vi "Define DataTable Columns.vi"(8 "error in (no error)":errorcluster, 9 "ReadOnly":bool, 10 "ColumnSetup":T1[](array[typedef]) {"MinWidth" min=2 step=1; "AutoSizeMode" items=["None"=1, "ColumnHeader"=2, "AllCellsExceptHeader"=4, "AllCells"=6, "DisplayedCellsExceptHeader"=8, "DisplayedCells"=10, "Fill"=16]; "FillWeight" min=1 max=100}, 11 "DataTable In":refnum<class "DataTable.lvclass">) -> (0 "error out":errorcluster, 3 "DataTable Out":refnum<class "DataTable.lvclass">)   [LabVIEW 2020, in "DataGrid.lvlib" / "DataTable.lvclass"]
doc: "Defines the columns of the dataTable that is used to store all display data. If called more than once, it will add columns to the existing dataTable, so resulting in more (possibly duplicate) columns."
uses:
  DataTable/DataTable.lvclass
  GridColumn/ColumnDefinition.ctl
  GridColumn/ColumnType.ctl
  DataTable/DataTable.lvclass/DataTable.ctl
  System.Data
  DataTable/Read DataTable.vi
  GridColumn/GridColumn.lvclass
panel:
  out "fl":bool
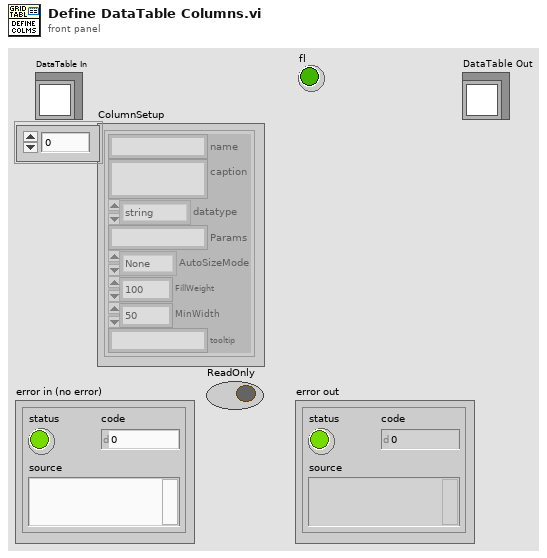
[diagram p1: front panel]
types:
  T1 = typedef "DataGrid.lvlib/GridColumn.lvclass/ColumnDefinition.ctl" = cluster{"name":string, "caption":string, "datatype":T2, "Params":string, "AutoSizeMode":i32, "FillWeight":sgl, "MinWidth":u32, "tooltip":string}
  T2 = typedef "DataGrid.lvlib/GridColumn.lvclass/ColumnType.ctl" = enum16{"string", "image", "check", "numeric", "timestamp", "button", "combo", "link"}
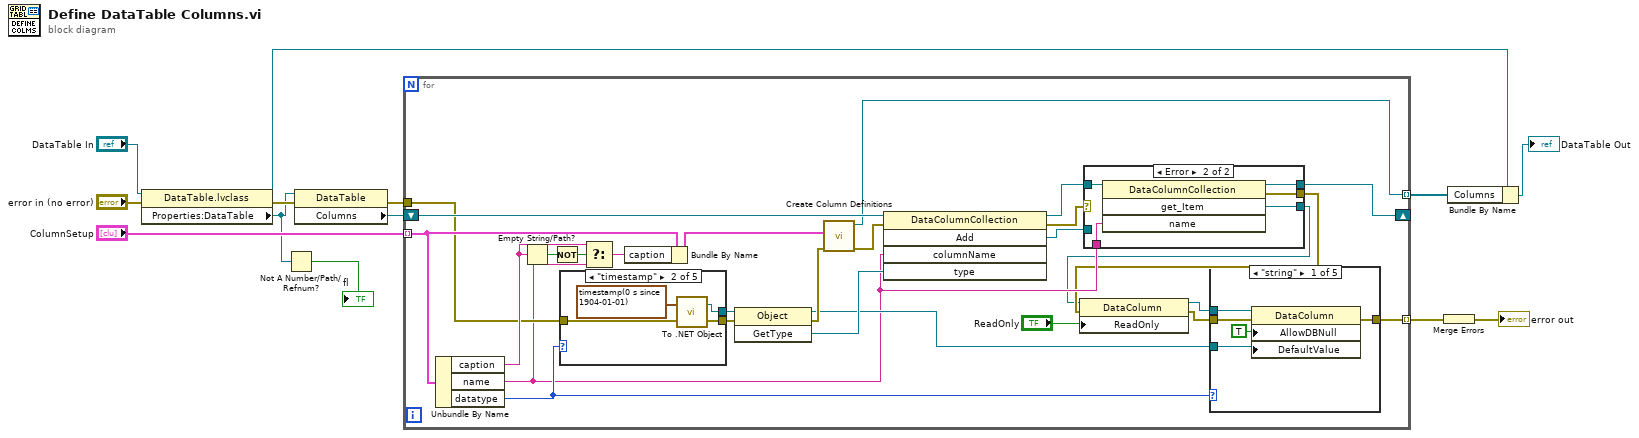
[diagram p0: block diagram]
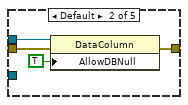
[diagram p3: hidden frame]
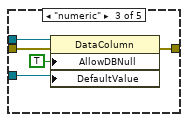
[diagram p4: hidden frame]
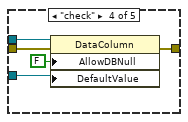
[diagram p5: hidden frame]
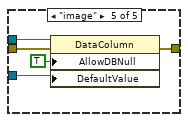
[diagram p6: hidden frame]
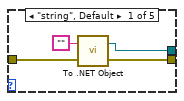
[diagram p7: hidden frame]
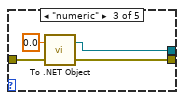
[diagram p8: hidden frame]
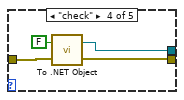
[diagram p9: hidden frame]
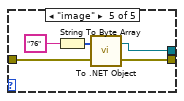
[diagram p10: hidden frame]
diagram:
  n1 = property class="DataTable.lvclass"(reference="DataTable In", error in="error in (no error)") -> (reference out=w8:refnum<class "DataTable.lvclass">, error out=w4:errorcluster, "Properties:DataTable"=w2:refnum<k24>)
  n2 = Not A Number/Path/Refnum?(number/path/refnum=w2) -> (NaN/Path/Refnum?=→"fl":bool)
  n3 = property class="DataTable"(reference=w2, error in=w4) -> (error out=w3:errorcluster, "Columns"=w10:refnum<k24>)  [unwired: 1 out]
  n4 = for {
    tunnel: "ColumnSetup" -> [w35] mode=indexing
    tunnel: [w40] -> w11 mode=indexing
    shift-right: [w16] -> _
    shift-left: w10 -> [w39]
    tunnel: [w38] -> w6 mode=indexing
    tunnel: w3 -> [w23]
    n5 = Unbundle By Name(w35) -> ("caption"=w33:string, "name"=w20:string, "datatype"=w22:T2)
    n6 = Empty String/Path?(string/path=w33) -> (empty?=w37:bool)
    n7 = Not(x=w37) -> (.not. x?=w24:bool)
    n8 = case shown="\"timestamp\"" w22 {
      tunnel: [w75 w79 w83 w87 w91] -> w31
      tunnel: [w74 w78 w82 w86 w90] -> w29
      tunnel: w23 -> [w73 w77 w81 w85 w89]
      frame "string", Default {
        n9 = call <vilib>:"To .NET Object.vi"("error in (no error)"=w73, "anything"="" ("name")) -> ("error out"=w74:errorcluster, ".NET object"=w75:refnum<k24>)
      }
      frame "timestamp" {
        n10 = call <vilib>:"To .NET Object.vi"("error in (no error)"=w77, "anything"=timestamp(0 s since 1904-01-01) ("name")) -> ("error out"=w78:errorcluster, ".NET object"=w79:refnum<k24>)
      }
      frame "numeric" {
        n11 = call <vilib>:"To .NET Object.vi"("error in (no error)"=w81, "anything"=0.0 ("name")) -> ("error out"=w82:errorcluster, ".NET object"=w83:refnum<k24>)
      }
      frame "check" {
        n12 = call <vilib>:"To .NET Object.vi"("error in (no error)"=w85, "anything"=FALSE) -> ("error out"=w86:errorcluster, ".NET object"=w87:refnum<k24>)
      }
      frame "image" {
        n13 = String To Byte Array(string="76") -> (unsigned byte array=w93:u8[])
        n14 = call <vilib>:"To .NET Object.vi"("error in (no error)"=w89, "anything"=w93) -> ("error out"=w90:errorcluster, ".NET object"=w91:refnum<k24>)
      }
    }
    n15 = Select(t=w33, s=w24, f=w20) -> (s? t:f=w36:string)
    n16 = Bundle By Name(cluster=w35, "caption"=w36) -> (w34:T1)
    n17 = invoke class="Object" method="GetType"(reference=w31, error in=w29) -> (reference out=w25:refnum<k24>, error out=w28:errorcluster, "GetType"=w30:refnum<k24>)  [unwired: 1 in]
    n18 = call "Create Column Definitions.vi"("error in (no error)"=w28, "Column"=w34) -> ("error out"=w21:errorcluster, "GridColumn out"=w38:refnum<class "GridColumn.lvclass">)  [unwired: 8 in]
    n19 = invoke class="DataColumnCollection" method="Add"(reference=w39, error in=w21, "columnName"=w20, "type"=w30) -> (reference out=w17:refnum<k24>, error out=w19:errorcluster, "Add"=w15:refnum<k24>)  [unwired: 1 in, 2 out]
    n20 = case shown="Error" w19 {
      selector: w19 -> [w43 _]
      tunnel: w17 -> [w41 w48]
      tunnel: [w42 w47] -> w14
      tunnel: w20 -> [_ w46]
      tunnel: [w43 w45] -> w18
      tunnel: [w41 w44] -> w16
      tunnel: w15 -> [w42 _]
      frame No Error {
      }
      frame Error {
        n21 = invoke class="DataColumnCollection" method="get_Item"(reference=w48, "name"=w46) -> (reference out=w44:refnum<k24>, error out=w45:errorcluster, "get_Item"=w47:refnum<k24>)  [unwired: 2 in, 1 out]
      }
    }
    n22 = property class="DataColumn"(reference=w14, error in=w18, "ReadOnly"="ReadOnly") -> (reference out=w27:refnum<k24>, error out=w26:errorcluster)
    n23 = case shown="\"string\"" w22 {
      tunnel: w27 -> [w51 w55 w60 w65 w70]
      tunnel: w26 -> [w53 w57 w62 w67 w72]
      tunnel: [w52 w56 w61 w66 w71] -> w40
      tunnel: w25 -> [w49 _ w58 w63 w68]
      frame "string" {
        n24 = property class="DataColumn"(reference=w51, error in=w53, "AllowDBNull"=TRUE, "DefaultValue"=w49) -> (error out=w52:errorcluster)  [unwired: 1 out]
      }
      frame Default {
        n25 = property class="DataColumn"(reference=w55, error in=w57, "AllowDBNull"=TRUE) -> (error out=w56:errorcluster)  [unwired: 1 out]
      }
      frame "numeric" {
        n26 = property class="DataColumn"(reference=w60, error in=w62, "AllowDBNull"=TRUE, "DefaultValue"=w58) -> (error out=w61:errorcluster)  [unwired: 1 out]
      }
      frame "check" {
        n27 = property class="DataColumn"(reference=w65, error in=w67, "AllowDBNull"=FALSE, "DefaultValue"=w63) -> (error out=w66:errorcluster)  [unwired: 1 out]
      }
      frame "image" {
        n28 = property class="DataColumn"(reference=w70, error in=w72, "AllowDBNull"=TRUE, "DefaultValue"=w68) -> (error out=w71:errorcluster)  [unwired: 1 out]
      }
    }
  }
  n29 = Merge Errors(w11) -> (→"error out":errorcluster)
  n30 = Bundle By Name(cluster=w8, "Columns"=w6) -> (→"DataTable Out":refnum<class "DataTable.lvclass">)
